vi "DSF.Engine.Plugin.Transfer.Parse.vi"(8 "error in (no error)":errorcluster, 10 "Transfer":refnum<class "DSF.Engine.Transfer.lvclass">, 11 "Plugin in":refnum<class "DSF.Engine.Plugin.lvclass">) -> (0 "error out":errorcluster, 3 "Plugin out":refnum<class "DSF.Engine.Plugin.lvclass">)   [LabVIEW 2017, in "DSF.Engine.lvlib" / "DSF.Engine.Plugin.lvclass"]
uses:
  DSF.Engine.Plugin.lvclass
  Transfer/DSF.Engine.Transfer.lvclass
  DSF.Engine.Plugin.lvclass/DSF.Engine.Plugin.ctl
  Transfer/DSF.Engine.Transfer.lvclass/DSF.Engine.Transfer.ctl
  Shared/Classes/Transfer/DSF.Shared.Configuration.Transfer.lvclass/DSF.Shared.Configuration.Transfer.ctl
  Shared/Classes/Transfer/DSF.Shared.Configuration.Transfer.lvclass
  Buffer/DSF.Engine.Memory.Buffer.lvclass
  Pointer/DSF.Engine.Pointer.DBL.lvclass
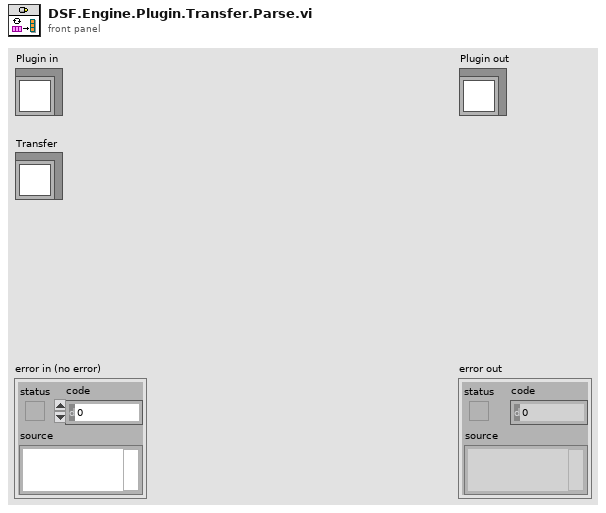
[diagram p1: front panel]
types:
  T1 = typedef "DSF.Engine.lvlib/DSF.Engine.Typedefs.Type Buffers.ctl" = cluster{"Bool":bool[], "SGL":sgl[], "DBL":dbl[], "I8":i8[], "I16":i16[], "I32":i32[], "I64":i64[], "U8":u8[], "U16":u16[], "U32":u32[], "U64":u64[]}
  T2 = typedef "DSF.Shared.lvlib/DSF.Shared.Typedefs.Configuration.Transfer.Channel Block Descriptor.ctl" = cluster{"First Channel Descriptor":T3, "count":u64, "vs channel index":u64}
  T3 = typedef "DSF.Shared.lvlib/DSF.Shared.Typedefs.Configuration.Transfer.Channel Descriptor.ctl" = cluster{"Channel Parameters":T4, "VS Channel Ref":T6}
  T4 = typedef "DSF.Shared.lvlib/DSF.Shared.Typedefs.Configuration.Transfer.Channel Parameters.ctl" = cluster{"offset":u64, "data type":T5}
  T5 = typedef "DSF.Shared.lvlib/DSF.Shared.Typedefs.Data Type.ctl" = enum8{"Bool", "SGL", "DBL", "I8", "I16", "I32", "I64", "U8", "U16", "U32", "U64"}
  T6 = typedef "Custom Device API.lvlib/Custom Device Item Ref.ctl" = u64
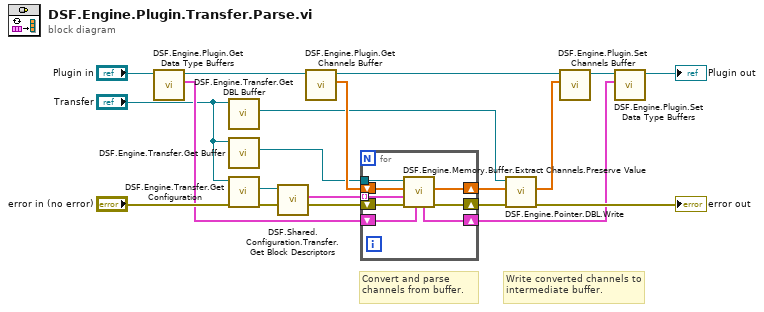
[diagram p0: block diagram]
diagram:
  # "Write converted channels to intermediate buffer."
  # "Convert and parse channels from buffer."
  n1 = call "DSF.Engine.Plugin.Get Data Type Buffers.vi"("Plugin in"="Plugin in") -> ("data type buffers"=w8:T1, "Plugin out"=w11:refnum<class "DSF.Engine.Plugin.lvclass">)  [unwired: 9 in]
  n2 = call "DSF.Engine.Transfer.Get DBL Buffer.vi"("Transfer in"="Transfer") -> ("DBL Buffer"=w4:refnum<class "DSF.Engine.Pointer.DBL.lvclass">)  [unwired: 9 in, 1 out]
  n3 = call "DSF.Engine.Transfer.Get Buffer.vi"("Transfer in"="Transfer") -> ("Buffer"=w15:refnum<class "DSF.Engine.Memory.Buffer.lvclass">)  [unwired: 9 in, 1 out]
  n4 = call "DSF.Engine.Transfer.Get Configuration.vi"("Transfer in"="Transfer") -> ("Configuration"=w16:refnum<class "DSF.Shared.Configuration.Transfer.lvclass">)  [unwired: 9 in, 1 out]
  n5 = call "DSF.Shared.Configuration.Transfer.Get Block Descriptors.vi"("Transfer Configuration in"=w16) -> ("Channel Blocks"=w14:T2[])  [unwired: 9 in, 1 out]
  n6 = call "DSF.Engine.Plugin.Get Channels Buffer.vi"("Plugin in"=w11) -> ("channels buffer"=w18:dbl[], "Plugin out"=w13:refnum<class "DSF.Engine.Plugin.lvclass">)  [unwired: 9 in]
  n7 = for {
    shift-right: [w25] -> w5
    shift-left: w18 -> [w22]
    shift-right: [w26] -> w6
    shift-left: "error in (no error)" -> [w24]
    tunnel: w15 -> [w21]
    tunnel: w14 -> [w23] mode=indexing
    shift-right: [w20] -> w1
    shift-left: w8 -> [w19]
    n8 = call "DSF.Engine.Memory.Buffer.Extract Channels.Preserve Value.vi"("Data Type Buffers in"=w19, "error in (no error)"=w24, "Channel Block"=w23, "VS Channels Array in"=w22, "Buffer in"=w21) -> ("error out"=w26:errorcluster, "VS Channels Array out"=w25:dbl[], "Data Type Buffers out"=w20:T1)  [unwired: 3 in, 1 out]
  }
  n9 = call "DSF.Engine.Pointer.DBL.Write.vi"("error in (no error)"=w6, "buffer in"=w5, "DBL Pointer in"=w4) -> ("error out"=→"error out":errorcluster, "buffer out"=w3:dbl[])  [unwired: 6 in, 1 out]
  n10 = call "DSF.Engine.Plugin.Set Channels Buffer.vi"("channels buffer"=w3, "Plugin in"=w13) -> ("Plugin out"=w10:refnum<class "DSF.Engine.Plugin.lvclass">)  [unwired: 9 in]
  n11 = call "DSF.Engine.Plugin.Set Data Type Buffers.vi"("data type buffers"=w1, "Plugin in"=w10) -> ("Plugin out"=→"Plugin out":refnum<class "DSF.Engine.Plugin.lvclass">)  [unwired: 9 in]
